vi "Offset Locking- Main with Slave Tracking v2.2.vi"() -> ()   [LabVIEW 2018]
uses:
  <vilib>/Utility/error.llb/DialogType.ctl
  <vilib>/Analysis/1siggen.llb/Ramp Pattern by Samples.vi
  <vilib>/measure/mamon.llb/Waveform Peak Detection for 1 Chan.vi
  <vilib>/addons/control/pid/pid.llb/PID Advanced (DBL).vi
  <vilib>/measure/NI_MAPro.lvlib
  <vilib>/addons/control/pid/NI_PID_pid.lvlib
  <vilib>/Analysis/NI_AALBase.lvlib
  <vilib>/measure/NI_MABase.lvlib
panel:
  in  "width":i32=1000
  in  "start":dbl format="%0.2f"
  in  "end":dbl=1.0 format="%0.2f"
  in  "samples":i32=128
  in  "Waveform Test?":bool
  in  "reset signal":bool
  in  "phase":dbl format="%.2p"
  out "Chirp Rate":dbl format="%#_g GHz/ms"
  out "Single Mode?":bool
  out "# of Peaks found when Chirping?":i32
  in  "Minimum amplitude for Slave":dbl=0.15 format="%.2p"
  in  "Minimum \namplitude\nfor peaks":dbl=0.8 format="%#_13g V"
  in  "PZT Voltage to \nFrequency Conversion":dbl=-1.41655 format="%#_g V/GHz"
  out "PZT Chirp Output":waveform(dbl)(graph)
  in  "offset":dbl format="%0.2p V"
  in  "Sampling Info":cluster{"Fs":dbl, "#s":dbl}={"Fs"=10000.0, "#s"=100.0} {"Fs" format="%.2p"}
  in  "frequency":dbl=10.0 format="%0.2p Hz"
  in  "Chirp Amplitude":dbl=1.5 format="%0.2p GHz"
  in  "Run Chirp Program?":bool
  out "Run Time (min)":dbl
  out "standard deviation":dbl format="%0.3e"
  in  "Ref Peak 2":i32=2
  in  "Ref Peak":i32=3
  in  "First Cal Peak":i32=2
  in  "Last Cal Peak":i32=4
  out "# found":i32
  out "Offset":dbl(graph)
  in  "Manual PZT Control":dbl format="%#_g V"
  in  "Engage PZT PID?":bool
  out "Offset (GHz)":dbl format="%#_4g"
  in  "# of Shots for Averaging":i32=100
  in  "Name Convention":string="Chirp Offset Lock Log"
  in  "Save Directory":path=path "C:/Users/LabUser/Google Drive/Measurements/04-2018"
  out "Four peaks?":bool
  out "PZT Output":dbl(graph)
  in  "PID Gains":T1={"proportional gain (Kc)"=-1.0, "integral time (Ti, min)"=0.01, "derivative time (Td, min)"=0.0} {"derivative time (Td, min)" format="%.3f"; "integral time (Ti, min)" format="%.3f"; "proportional gain (Kc)" format="%.3f"}
  out "dt out (s)":dbl format="%.3f"
  in  "Frequency Offset Setpoint (GHz)":dbl=7.79 format="%.3f"
  out "GHz/sec":dbl
  out "dt":dbl format="%#_4g"
  out "Locations":dbl[](array[numeric]) format="%.2p"
  out "Amplitudes":dbl[](array[numeric]) format="%.2p"
  out "2nd Derivatives":dbl[](array[numeric]) format="%.2p"
  out "10 GHz FPI":dynamicdata(graph)
  in  "Stop":bool
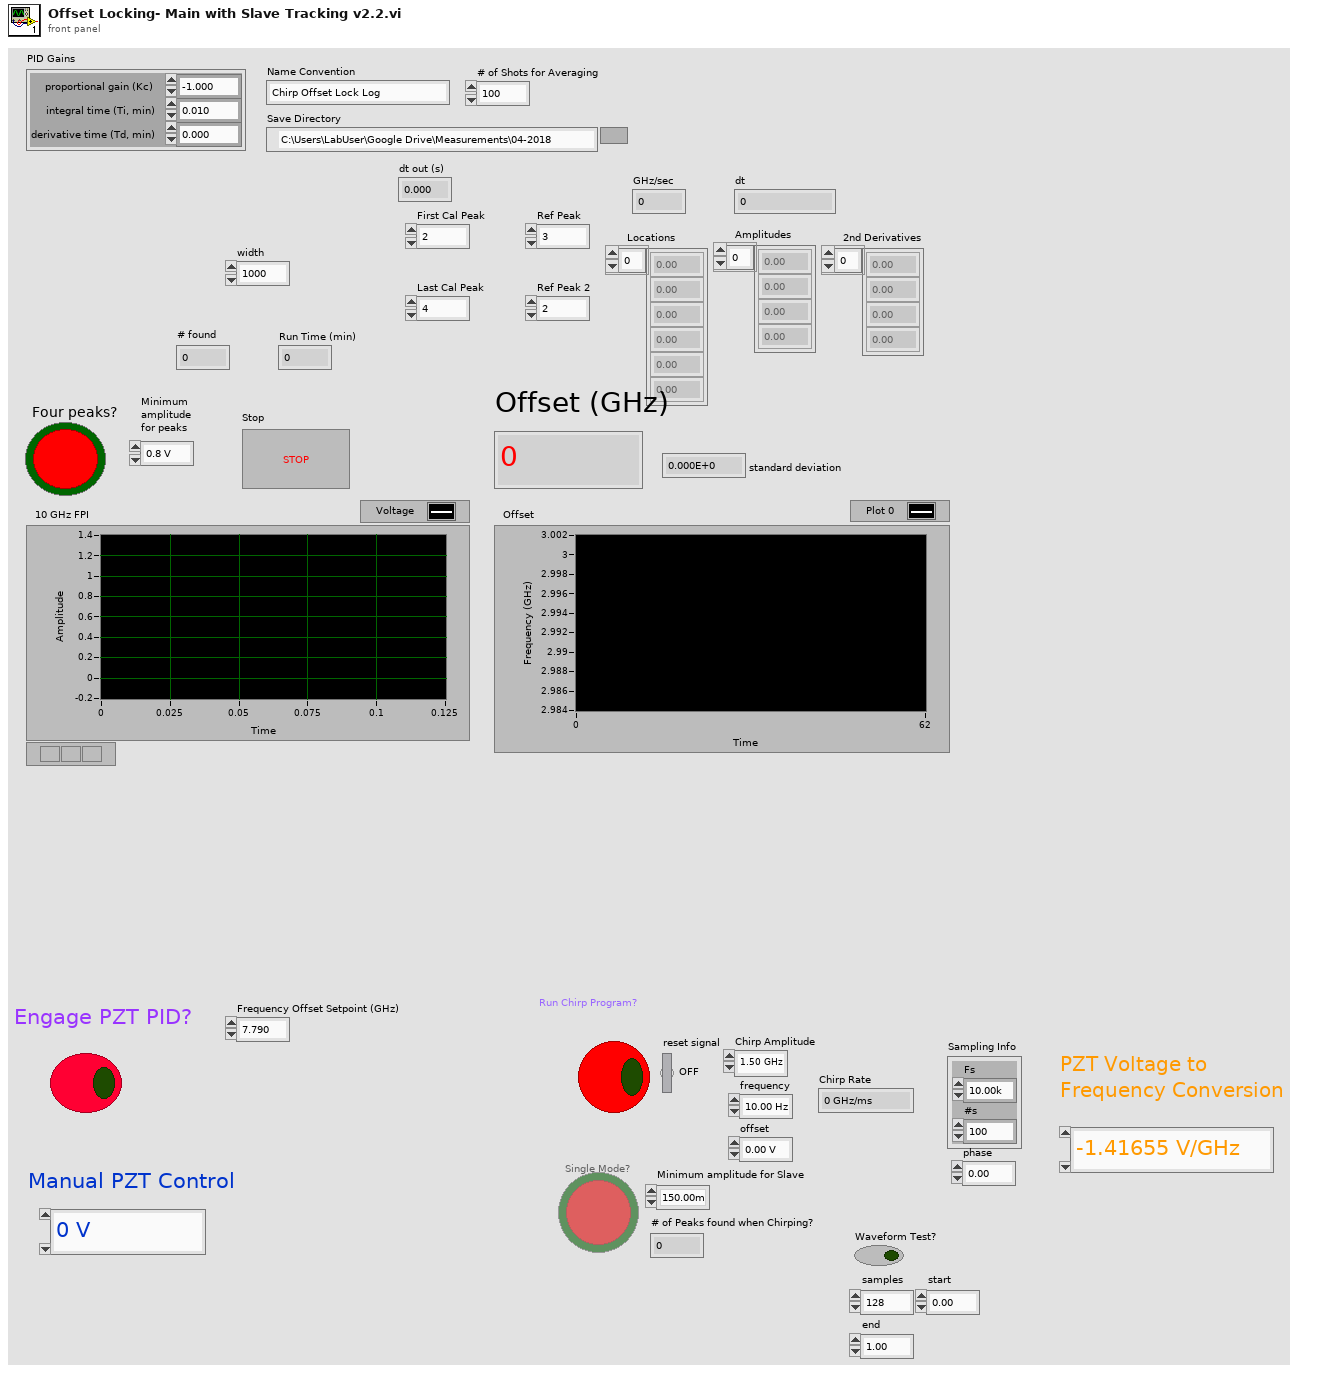
[diagram p1: front panel]
types:
  T1 = cluster{"proportional gain (Kc)":dbl, "integral time (Ti, min)":dbl, "derivative time (Td, min)":dbl}
  T2 = enum8{"Enabled", "Disabled", "Disabled and Grayed Out"}
  T3 = typedef "DialogType.ctl" = u16
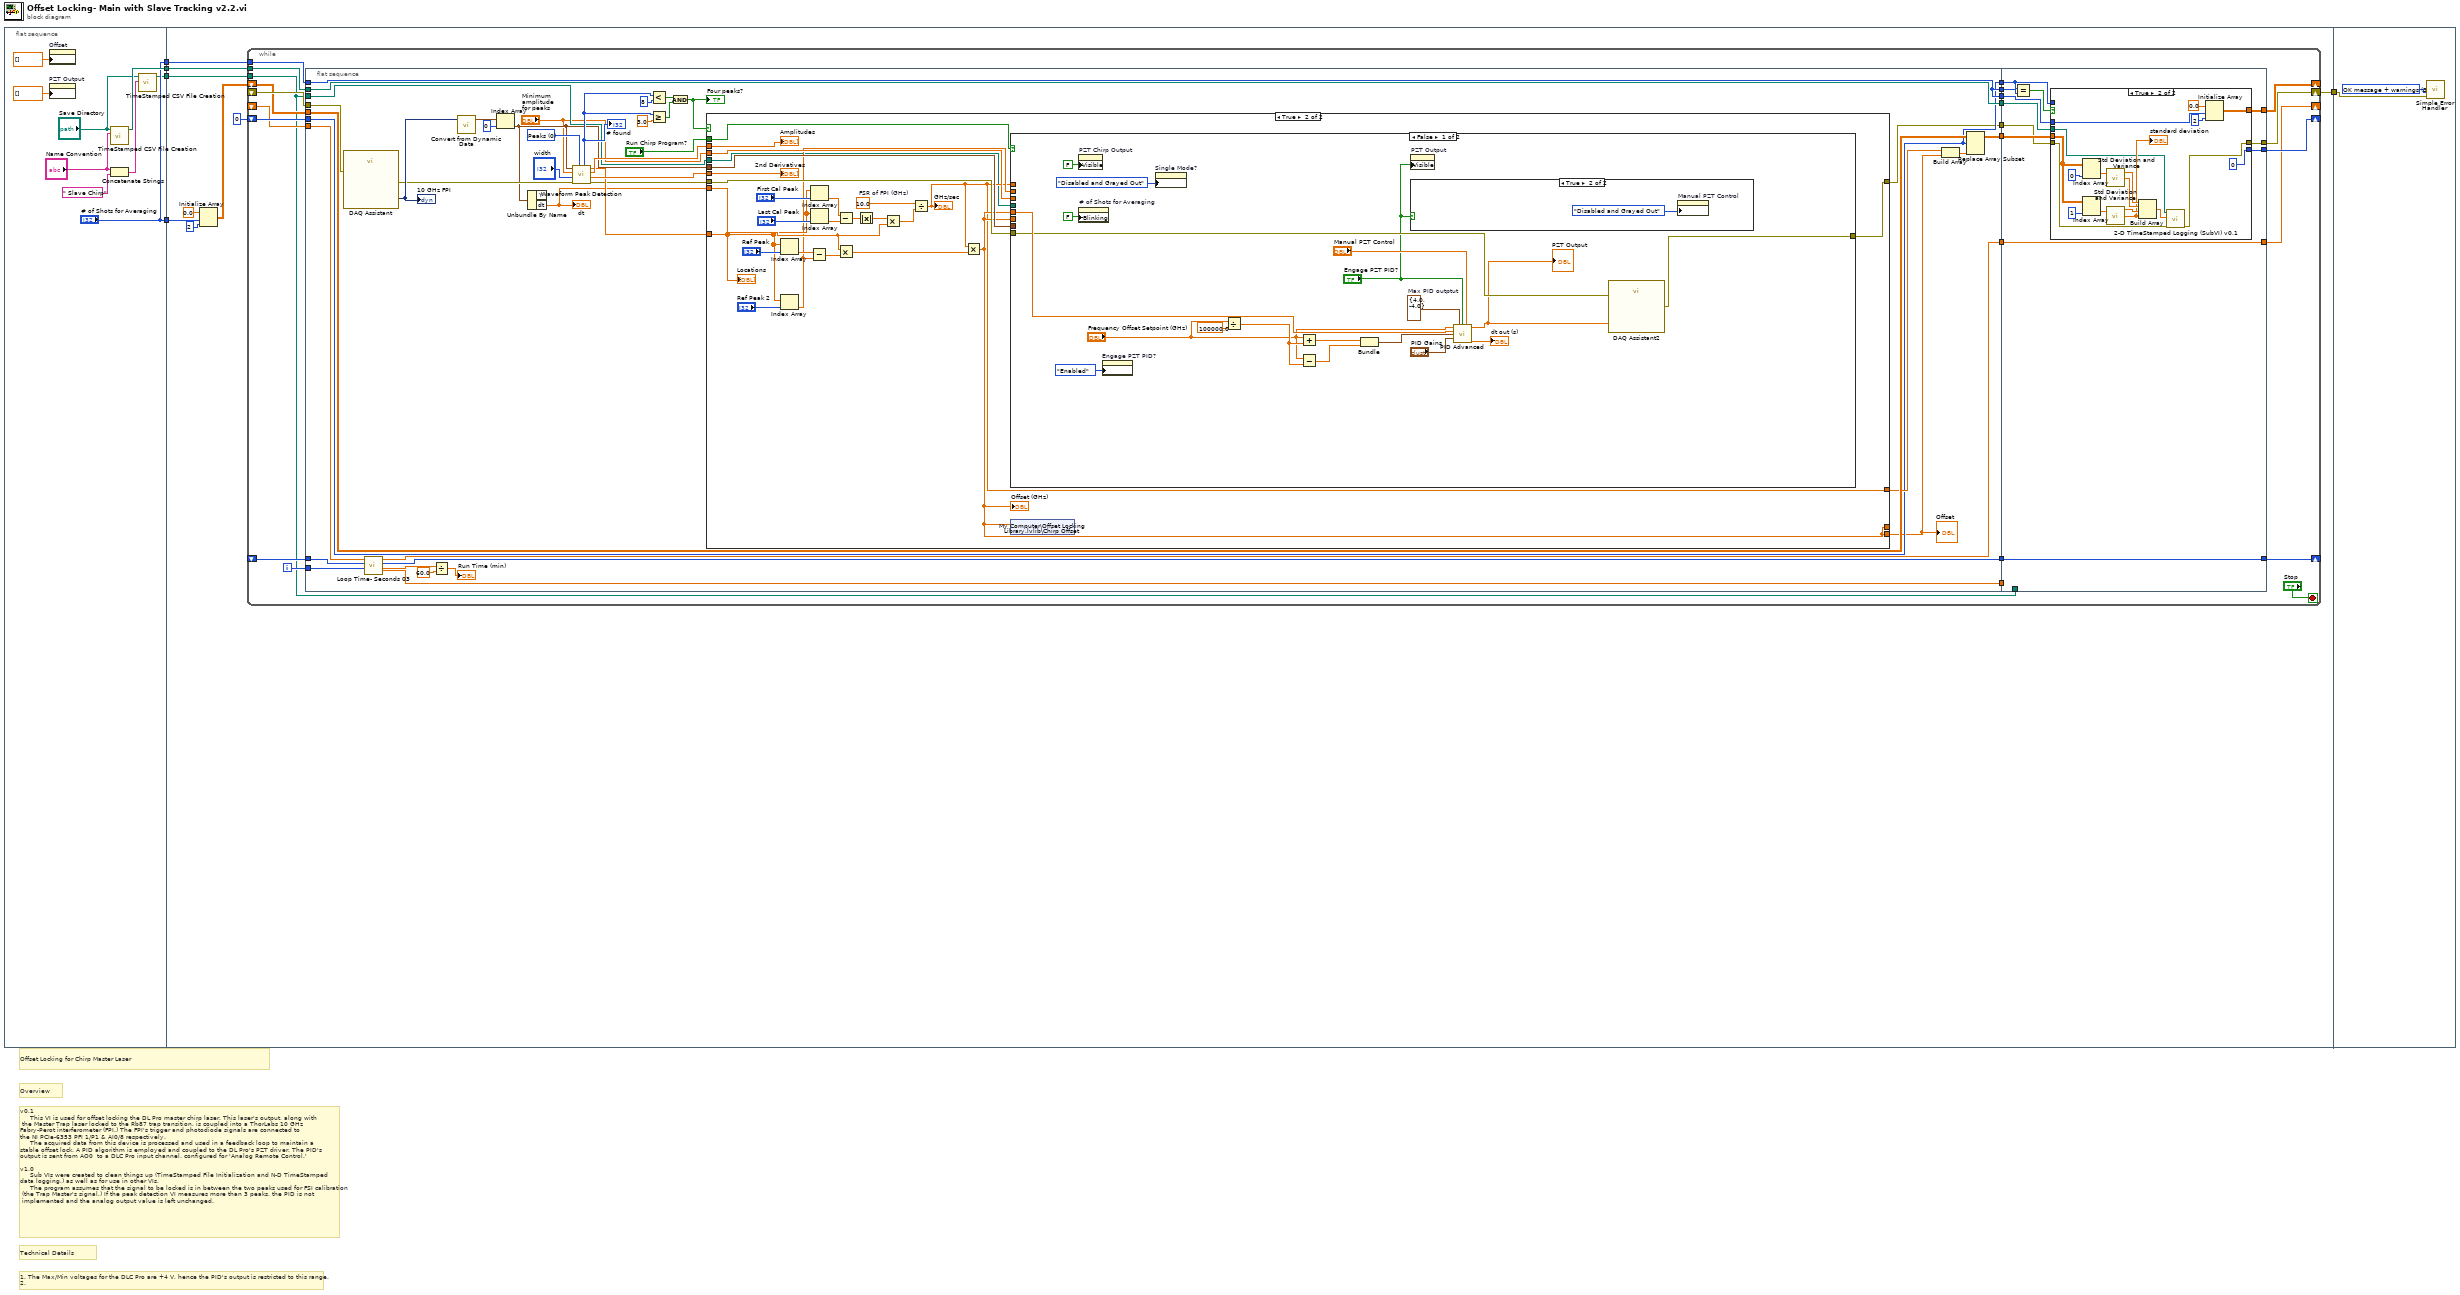
[diagram p0: block diagram]
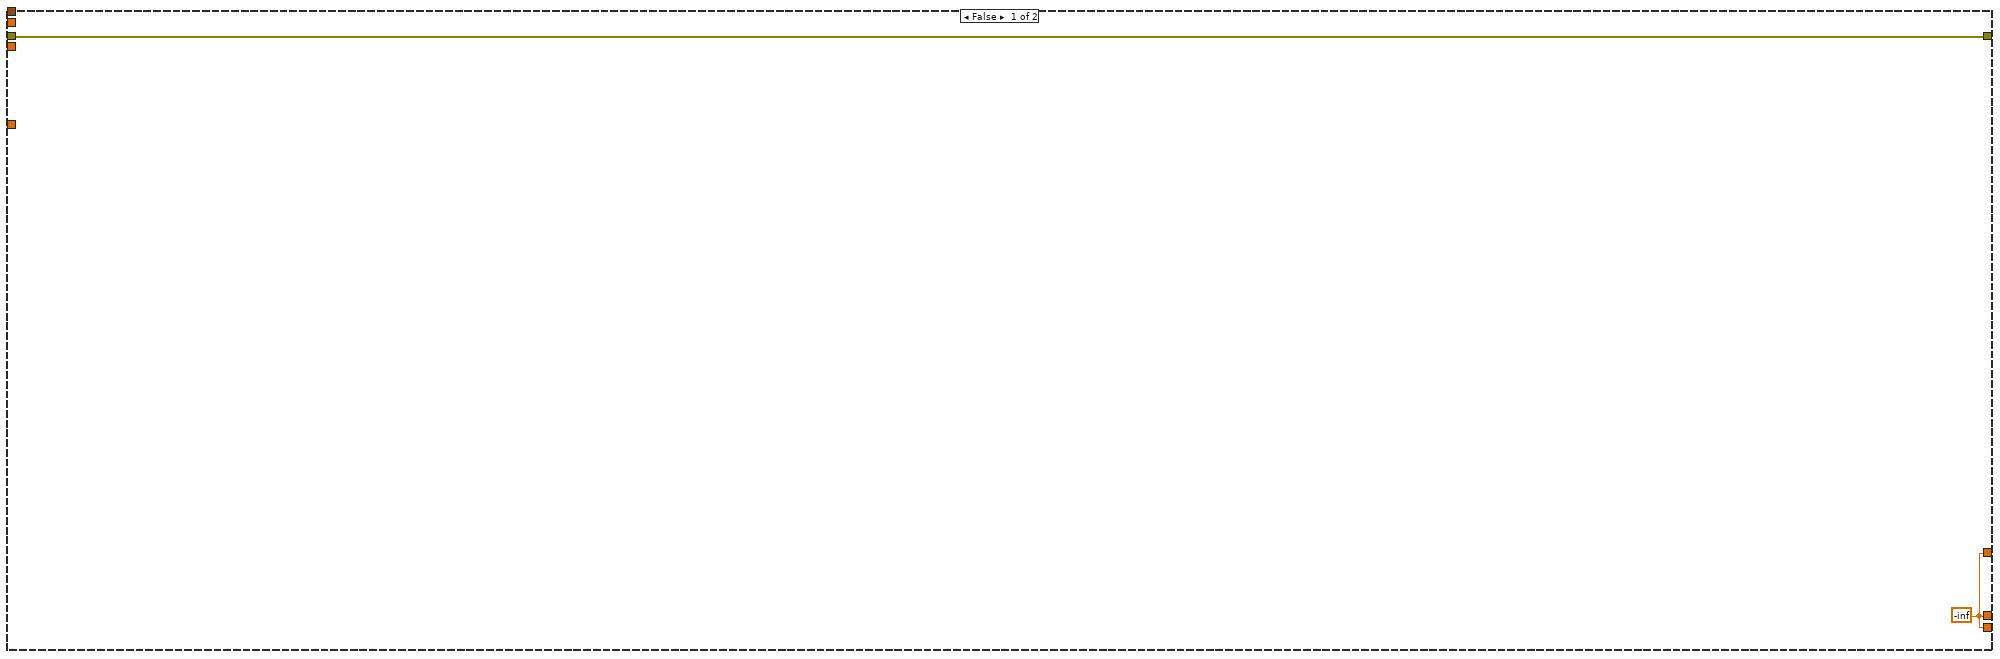
[diagram p2: hidden frame]
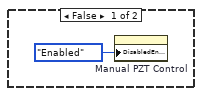
[diagram p3: hidden frame]
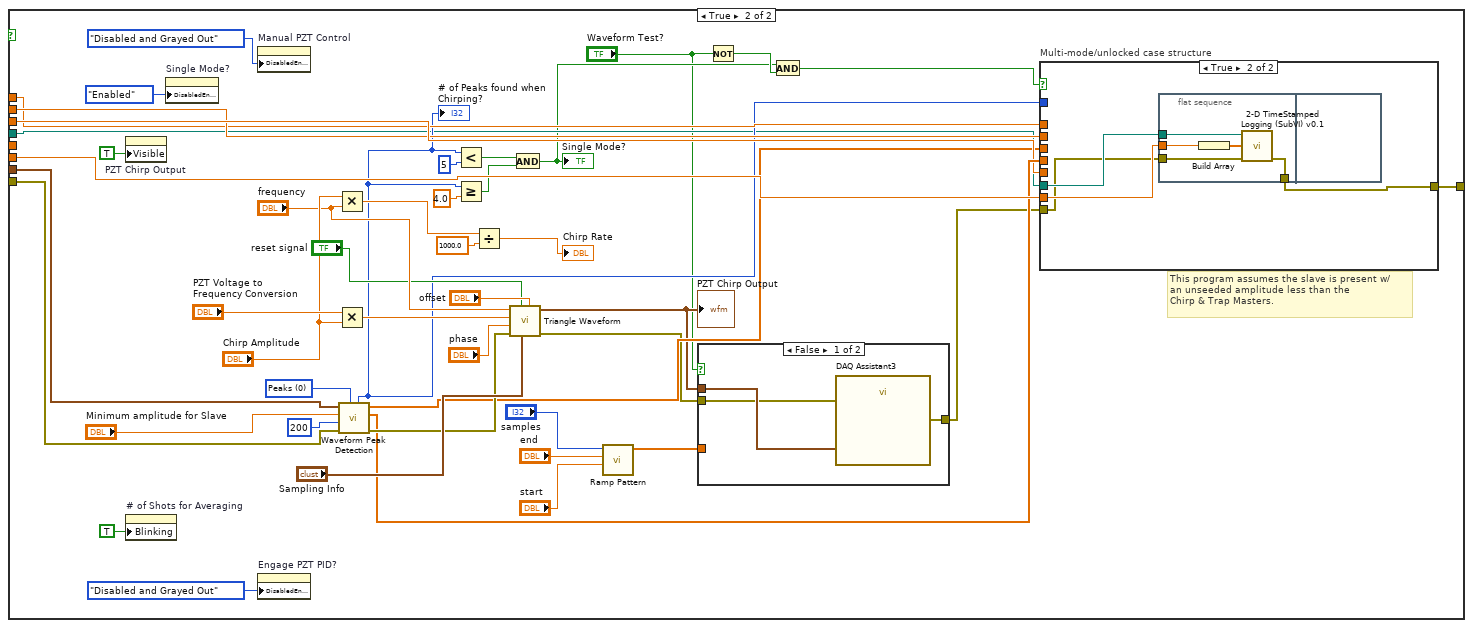
[diagram p4: hidden frame]
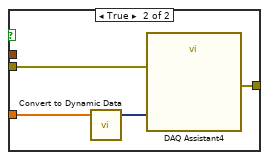
[diagram p5: hidden frame]
diagram:
  # "1. The Max/Min voltages for the DLC Pro are +4 V, hence the PID's output is restricted to this range.\n2."
  # "Technical Details"
  # "v0.1\n     This VI is used for offset locking the DL Pro master chirp laser. This laser's output, along with\n the Master Trap laser locked to the Rb87 trap transition, is coupled into a ThorLabs 10 GHz \nFabry-Perot interferometer (FPI.) The FPI's trigger and photodiode signals are connected to \nthe NI PCIe-6353 PFI 1/P1 & AI0/8 respectively. \n     The acquired data from this device is processed and used in a feedback loop to maintain a \nstable offset lock. A PID algorithm is employed and coupled to the DL Pro's PZT driver. The PID's\noutput is sent from AO0  to a DLC Pro input channel, configured for 'Analog Remote Control.'\n\nv1.0\n     Sub VIs were created to clean things up (TimeStamped File Initialization and N-D TimeStamped \ndata logging,) as well as for use in other VIs.\n     The program assumes that the signal to be locked is in between the two peaks used for FSI calibration\n (the Trap Master's signal.) If the peak detection VI measures more than 3 peaks, the PID is not\n implemented and the analog output value is left unchanged."
  # "Overview"
  # "Offset Locking for Chirp Master Laser"
  n1 = flat-sequence {
    tunnel: [w14] -> w5
    tunnel: ["# of Shots for Averaging"] -> w3
    tunnel: ["# of Shots for Averaging"] -> w2
    tunnel: [w6] -> w1
    tunnel: w5 -> [w23]
    tunnel: [w22] -> w4
    tunnel: w3 -> [w20]
    tunnel: w2 -> [w17]
    tunnel: w1 -> [w15]
    tunnel: w4 -> [w238]
    frame #0 {
      n2 = property on="Offset" class="WFChart (strict)"("History Data"=dbl[] []) -> ()  [unwired: 2 in, 2 out]
      n3 = property on="PZT Output" class="WFChart (strict)"("History Data"=dbl[] []) -> ()  [unwired: 2 in, 2 out]
      n4 = call "TimeStamped CSV File Creation.vi"("Name Convention"="Name Convention", "Save Directory"="Save Directory") -> ("path"=w14:path)  [unwired: 8 in, 1 out]
      n5 = Concatenate Strings("Name Convention", " Slave Chirp" ("string")) -> (w8:string)
      n6 = call "TimeStamped CSV File Creation.vi"("Name Convention"=w8, "Save Directory"="Save Directory") -> ("path"=w6:path)  [unwired: 8 in, 1 out]
    }
    frame #1 {
      n7 = Initialize Array(0.0 ("element"), w17, 2 ("dimension size")) -> (w19:dbl[][])
      n8 = while {
        shift-right: [w35] -> w22
        shift-left: _ -> [w46]
        tunnel: w23 -> [w44]
        shift-right: [w33] -> _
        shift-left: 0 -> [w42]
        tunnel: w20 -> [w40]
        shift-right: [w34] -> _
        shift-left: w19 -> [w37]
        shift-right: [w31] -> _
        shift-left: _ -> [w28]
        shift-right: [w29] -> _
        shift-left: _ -> [w27]
        tunnel: w15 -> [w24]
        i -> [w26]
        stop <- "Stop" stop-if-true
        n9 = flat-sequence {
          tunnel: w46 -> [w77]
          tunnel: [w53] -> w45
          tunnel: w44 -> [w75]
          tunnel: [w75] -> w43
          tunnel: w42 -> [w69]
          tunnel: [w69] -> w41
          tunnel: w40 -> [w70]
          tunnel: [w70] -> w39
          tunnel: [w74] -> w38
          tunnel: w37 -> [w73]
          tunnel: [w70] -> w36
          tunnel: [w68] -> w32
          tunnel: [w67] -> w30
          tunnel: w28 -> [w66]
          tunnel: w27 -> [w65]
          tunnel: w26 -> [w64]
          tunnel: [w56] -> w25
          tunnel: w24 -> [w50]
          tunnel: w45 -> [w211]
          tunnel: w43 -> [w212]
          tunnel: w41 -> [w206]
          tunnel: w39 -> [w216]
          tunnel: w38 -> [w213]
          tunnel: w36 -> [w214]
          tunnel: [w205] -> w35
          tunnel: [w210] -> w34
          tunnel: [w209] -> w33
          tunnel: w32 -> [w208]
          tunnel: [w208] -> w31
          tunnel: [w207] -> w29
          tunnel: w30 -> [w207]
          tunnel: w25 -> [_]
          tunnel: w24 -> [_]
          frame #0 {
            w79 = u16 0 items=["Peaks", "Valleys"] ("peaks/valleys")
            n10 = call "DAQ Assistant"("error in"=w77) -> ("data"=w84:dynamicdata, "error out"=w76:errorcluster)  [unwired: 16 in, 1 out]
            "10 GHz FPI" <- w84
            n11 = call "Loop Time- Seconds 03.vi"("Loop Iteration"=w64, "Shift Registered Time In"=w65, "Shift Registered In"=w66) -> ("t"=w56:dbl, "Shift Registered Time Out"=w67:u32, "Shift Registered Out"=w68:dbl)  [unwired: 6 in]
            n12 = Divide(x=w56, y=60.0) -> (x/y=→"Run Time (min)":dbl)
            n13 = call "Convert from Dynamic Data"("Dynamic Data Type"=w84) -> ("Array of Waveform"=w86:waveform(dbl)[])  [unwired: 3 in]
            n14 = Index Array(array=w86, index=0) -> (element=w51:waveform(dbl))
            n15 = Unbundle By Name(w51) -> ("dt"=w80:dbl)  [unwired: 1 out]
            "dt" <- w80
            n16 = call-poly <vilib>:"Waveform Peak Detection.vi"("peaks/valleys"=w79, "error in"=w76, "width"="width", "threshold"="Minimum \namplitude\nfor peaks", "Signal In"=w51) -> ("error out"=w54:errorcluster, "2nd Derivatives"=w82:dbl[], "Amplitudes"=w83:dbl[], "Locations"=w81:dbl[], "# found"=w61:i32)  [unwired: 2 in]
            "# found" <- w61
            n17 = Less?(x=w61, y=8) -> (x < y?=w59:bool)
            n18 = Greater Or Equal?(x=w61, y=3.0) -> (x >= y?=w62:bool)
            n19 = And(x=w59, y=w62) -> (x .and. y?=w58:bool)
            "Four peaks?" <- w58
            n20 = case shown="True" w58 {
              tunnel: w83 -> [_ w93]
              tunnel: w82 -> [_ w114]
              tunnel: w81 -> [_ w99]
              tunnel: w80 -> [_ w105]
              tunnel: [w88 w90] -> w72
              tunnel: [w88 w94] -> w63
              tunnel: [w88 w94] -> _
              tunnel: w54 -> [w87 w98]
              tunnel: [w87 w97] -> w53
              tunnel: "Run Chirp Program?" -> [_ w96]
              tunnel: w51 -> [_ w95]
              tunnel: "Minimum \namplitude\nfor peaks" -> [_ w92]
              tunnel: w50 -> [_ w89]
              frame False {
                w88 = -inf
              }
              frame True {
                w112 = 10.0  # FSR of FPI (GHz)
                n21 = Index Array(array=w99, index="Ref Peak") -> (element=w107:dbl)
                n22 = Index Array(array=w99, index="Ref Peak 2") -> (element=w91:dbl)
                n23 = Subtract(x=w107, y=w91) -> (x-y=w106:dbl)
                n24 = Index Array(array=w99, index="First Cal Peak") -> (element=w108:dbl)
                n25 = Index Array(array=w99, index="Last Cal Peak") -> (element=w113:dbl)
                n26 = Subtract(x=w108, y=w113) -> (x-y=w110:dbl)
                n27 = Multiply(x=w105, y=w106) -> (x*y=w104:dbl)
                n28 = Absolute Value(x=w110) -> (abs(x)=w109:dbl)
                n29 = Multiply(x=w109, y=w105) -> (x*y=w111:dbl)
                n30 = Divide(x=w112, y=w111) -> (x/y=w90:dbl)
                "GHz/sec" <- w90
                n31 = Multiply(x=w90, y=w104) -> (x*y=w94:dbl)
                "Offset (GHz)" <- w94
                n32 = case shown="False" w96 {
                  tunnel: w94 -> [w129 _]
                  tunnel: w98 -> [w128 w171]
                  tunnel: [w127 w144] -> w97
                  tunnel: w95 -> [_ w172]
                  tunnel: w94 -> [_ w168]
                  tunnel: w92 -> [_ w162]
                  tunnel: w91 -> [_ w160]
                  tunnel: w90 -> [_ w159]
                  tunnel: w89 -> [_ w146]
                  frame False {
                    w131 = cluster{"output high":dbl, "output low":dbl} {"output high"=4.0, "output low"=-4.0}  # Max PID outptut
                    n33 = property on="PZT Chirp Output" class="WFGraph (strict)"("Visible"=FALSE) -> ()  [unwired: 2 in, 2 out]
                    n34 = property on="# of Shots for Averaging" class="DigNum (strict)"("Blinking"=FALSE) -> ()  [unwired: 2 in, 2 out]
                    n35 = property on="Engage PZT PID?" class="Bool (strict)"("DisabledEnum"=T2."Enabled" ("Disabled")) -> ()  [unwired: 2 in, 2 out]
                    n36 = property on="Single Mode?" class="Bool (strict)"("DisabledEnum"=T2."Disabled and Grayed Out" ("Disabled")) -> ()  [unwired: 2 in, 2 out]
                    n37 = Divide(x="Frequency Offset Setpoint (GHz)", y=100000.0) -> (x/y=w119:dbl)
                    n38 = Add(x="Frequency Offset Setpoint (GHz)", y=w119) -> (x+y=w117:dbl)
                    n39 = Subtract(x="Frequency Offset Setpoint (GHz)", y=w119) -> (x-y=w116:dbl)
                    n40 = Bundle(w117, w116) -> (w115:cluster{dbl, dbl})  [unwired: 1 in]
                    n41 = property on="PZT Output" class="WFChart (strict)"("Visible"="Engage PZT PID?") -> ()  [unwired: 2 in, 2 out]
                    n42 = case shown="True" "Engage PZT PID?" {
                      frame False {
                        n43 = property on="Manual PZT Control" class="DigNum (strict)"("DisabledEnum"=T2."Enabled" ("Disabled")) -> ()  [unwired: 2 in, 2 out]
                      }
                      frame True {
                        n44 = property on="Manual PZT Control" class="DigNum (strict)"("DisabledEnum"=T2."Disabled and Grayed Out" ("Disabled")) -> ()  [unwired: 2 in, 2 out]
                      }
                    }
                    n45 = call-poly <vilib>:"PID Advanced.vi"("setpoint"="Frequency Offset Setpoint (GHz)", "output range"=w131, "auto? (T)"="Engage PZT PID?", "manual control"="Manual PZT Control", "process variable"=w129, "setpoint range"=w115, "PID gains"="PID Gains") -> ("output"=w126:dbl, "dt out (s)"=→"dt out (s)":dbl)  [unwired: 7 in]
                    "PZT Output" <- w126
                    n46 = call "DAQ Assistant2"("data"=w126, "error in"=w128) -> ("error out"=w127:errorcluster)  [unwired: 16 in, 1 out]
                  }
                  frame True {
                    w158 = u16 0 items=["Peaks", "Valleys"] ("peaks/valleys")
                    # "This program assumes the slave is present w/ \nan unseeded amplitude less than the \nChirp & Trap Masters."
                    n47 = property on="PZT Chirp Output" class="WFGraph (strict)"("Visible"=TRUE) -> ()  [unwired: 2 in, 2 out]
                    n48 = property on="# of Shots for Averaging" class="DigNum (strict)"("Blinking"=TRUE) -> ()  [unwired: 2 in, 2 out]
                    n49 = property on="Single Mode?" class="Bool (strict)"("DisabledEnum"=T2."Enabled" ("Disabled")) -> ()  [unwired: 2 in, 2 out]
                    n50 = property on="Manual PZT Control" class="DigNum (strict)"("DisabledEnum"=T2."Disabled and Grayed Out" ("Disabled")) -> ()  [unwired: 2 in, 2 out]
                    n51 = property on="Engage PZT PID?" class="Bool (strict)"("DisabledEnum"=T2."Disabled and Grayed Out" ("Disabled")) -> ()  [unwired: 2 in, 2 out]
                    n52 = Multiply(x="Chirp Amplitude", y="frequency") -> (x*y=w153:dbl)
                    n53 = Multiply(x="PZT Voltage to \nFrequency Conversion", y="Chirp Amplitude") -> (x*y=w174:dbl)
                    n54 = call-poly <vilib>:"Waveform Peak Detection.vi"("peaks/valleys"=w158, "error in"=w171, "width"=200, "threshold"="Minimum amplitude for Slave", "Signal In"=w172) -> ("error out"=w170:errorcluster, "Amplitudes"=w163:dbl[], "Locations"=w161:dbl[], "# found"=w147:i32)  [unwired: 2 in, 1 out]
                    "# of Peaks found when Chirping?" <- w147
                    n55 = Less?(x=w147, y=5) -> (x < y?=w164:bool)
                    n56 = Greater Or Equal?(x=w147, y=4.0) -> (x >= y?=w166:bool)
                    n57 = Divide(x=w153, y=1000.0) -> (x/y=→"Chirp Rate":dbl)
                    n58 = call <vilib>:"Triangle Waveform.vi"("offset"="offset", "sampling info"="Sampling Info", "reset signal"="reset signal", "error in (no error)"=w170, "phase"="phase", "amplitude"=w174, "frequency"="frequency") -> ("error out"=w148:errorcluster, "signal out"=w149:waveform(dbl))  [unwired: 3 in]
                    "PZT Chirp Output" <- w149
                    n59 = And(x=w164, y=w166) -> (x .and. y?=w142:bool)
                    "Single Mode?" <- w142
                    n60 = call-poly <vilib>:"Ramp Pattern.vi"("start"="start", "end"="end", "samples"="samples") -> ("Ramp Pattern"=w139:dbl[])  [unwired: 7 in, 1 out]
                    n61 = case shown="False" "Waveform Test?" {
                      tunnel: w149 -> [w184 _]
                      tunnel: w148 -> [w183 w188]
                      tunnel: [w182 w187] -> w145
                      tunnel: w139 -> [_ w186]
                      frame False {
                        n62 = call "DAQ Assistant3"("data"=w184, "error in"=w183) -> ("error out"=w182:errorcluster)  [unwired: 16 in, 1 out]
                      }
                      frame True {
                        n63 = call "Convert to Dynamic Data"("Array"=w186) -> ("Dynamic Data Type"=w185:dynamicdata)  [unwired: 3 in]
                        n64 = call "DAQ Assistant4"("data"=w185, "error in"=w188) -> ("error out"=w187:errorcluster)  [unwired: 16 in, 1 out]
                      }
                    }
                    n65 = Not(x="Waveform Test?") -> (.not. x?=w143:bool)
                    n66 = And(x=w142, y=w143) -> (x .and. y?=w141:bool)
                    n67 = case "Multi-mode/unlocked case structure" shown="True" w141 {
                      tunnel: w168 -> [_ w199]
                      tunnel: w147 -> [w195 _]
                      tunnel: w163 -> [w194 _]
                      tunnel: w162 -> [w193 _]
                      tunnel: w161 -> [w192 _]
                      tunnel: w160 -> [w191 _]
                      tunnel: w159 -> [w190 _]
                      tunnel: w146 -> [_ w198]
                      tunnel: w145 -> [w189 w197]
                      tunnel: [w189 w196] -> w144
                      frame False {
                        n68 = for {
                          N: w195 -> [_]
                          tunnel: w194 -> [_] mode=indexing
                          tunnel: w193 -> [_]
                          tunnel: w192 -> [_] mode=indexing
                          tunnel: w191 -> [_]
                          tunnel: w190 -> [_]
                        }
                      }
                      frame True {
                        n69 = flat-sequence {
                          tunnel: w199 -> [w204]
                          tunnel: w198 -> [w202]
                          tunnel: w197 -> [w201]
                          tunnel: [w200] -> w196
                          frame #0 {
                            n70 = Build Array(w204) -> (w203:dbl[])
                            n71 = call "2-D TimeStamped Logging (SubVI) v0.1.vi"("error in (no error)"=w201, "array"=w203, "path"=w202) -> ("error out"=w200:errorcluster)  [unwired: 8 in]
                          }
                          frame #1 {
                          }
                        }
                      }
                    }
                  }
                }
                n72 = shared-variable "My Computer\\Offset Locking Library.lvlib\\Chirp Offset"(w94) -> ()  [unwired: 1 in, 1 out]
                "2nd Derivatives" <- w114
                "Amplitudes" <- w93
                "Locations" <- w99
              }
            }
            "Offset" <- w63
            n73 = Build Array(w72, w63) -> (w71:dbl[])
            n74 = Replace Array Subset(array=w73, new element=w71, index (row)=w69) -> (w74:dbl[][])  [unwired: 1 in]
          }
          frame #1 {
            n75 = Equal?(x=w206, y=w216) -> (x = y?=w215:bool)
            n76 = case shown="True" w215 {
              tunnel: w214 -> [_ w220]
              tunnel: w213 -> [w219 w233]
              tunnel: w212 -> [_ w227]
              tunnel: w211 -> [w217 w226]
              tunnel: [w219 w223] -> w210
              tunnel: w206 -> [w218 _]
              tunnel: [w218 0] -> w209
              tunnel: [w217 w221] -> w205
              frame False {
              }
              frame True {
                n77 = Index Array(array=w233, index (col)=0 ("disabled index (col)")) -> (element=w236:dbl[])  [unwired: 1 in]
                n78 = Index Array(array=w233, index (col)=1 ("disabled index (col)")) -> (element=w234:dbl[])  [unwired: 1 in]
                n79 = call <vilib>:"Std Deviation and Variance.vi"("X"=w236) -> ("mean"=w232:dbl, "standard deviation"=w231:dbl)  [unwired: 1 in, 1 out]
                n80 = call <vilib>:"Std Deviation and Variance.vi"("X"=w234) -> ("mean"=w230:dbl, "standard deviation"=w229:dbl)  [unwired: 1 in, 1 out]
                "standard deviation" <- w229
                n81 = Build Array(w232, w231, w230, w229) -> (w228:dbl[])
                n82 = call "2-D TimeStamped Logging (SubVI) v0.1.vi"("error in (no error)"=w226, "array"=w228, "path"=w227) -> ("error out"=w221:errorcluster)  [unwired: 8 in]
                n83 = Initialize Array(0.0 ("element"), w220, 2 ("dimension size")) -> (w223:dbl[][])
              }
            }
          }
        }
      }
    }
    frame #2 {
      w239 = T3 3 items=["no dialog", "OK message", "continue or stop message", "OK message + warnings", "continue/stop + warnings"] ("type of dialog (OK msg:1)")
      n84 = call <vilib>:"Simple Error Handler.vi"("type of dialog (OK msg:1)"=w239, "error in (no error)"=w238) -> ()  [unwired: 3 in, 5 out]
    }
  }
